vi "List Project Contents.vi"(11 "Selected Project":refnum<vi>) -> (3 "Selected Project Out":refnum<vi>)   [LabVIEW 2014]
doc: "<b>Controls:</b> \n<b>Inputs:</b>\n<b>Exit:</b>\n\n\n<b>Save Data to File:</b>\n\n\n<b>Selected Project:</b>\n\n\n<b>Tab Control:</b>\n\n\n<b>Re-Scan:</b>\n\n\n<b>Outputs:</b>\n<b>Project Name:</b>\n\n\n<b>Progress:</b>\n\n\n<b>Selected Project 2:</b>\n\n\n<b>Project Description:</b>"
uses:
  <userlib>/GA/VI Documentation Tool/TYPE_Version Status.ctl
  <vilib>/Utility/miscctls.llb/LVRowAndColumnTypeDef.ctl
  Type Defs/TYPE_Sorted Project Items.ctl
  Type Defs/TYPE_Project Summary.ctl
panel:
  out "Project Name":string caption="Project\nName"
  out "Project Description":string caption="Project\nDescription"
  in  "Tab Control":T1(tab)
  out "Summary":T2
  in  "Items List":i32[](listbox)
  out "Progress":i32(slide) caption="Sorting Project Items By Location" max=35
  in  "Re-Scan":bool
  in  "Save Data to File":bool
  in  "Exit":bool
  # "User.lib VIs Summary"
  # "Project VIs Summary"
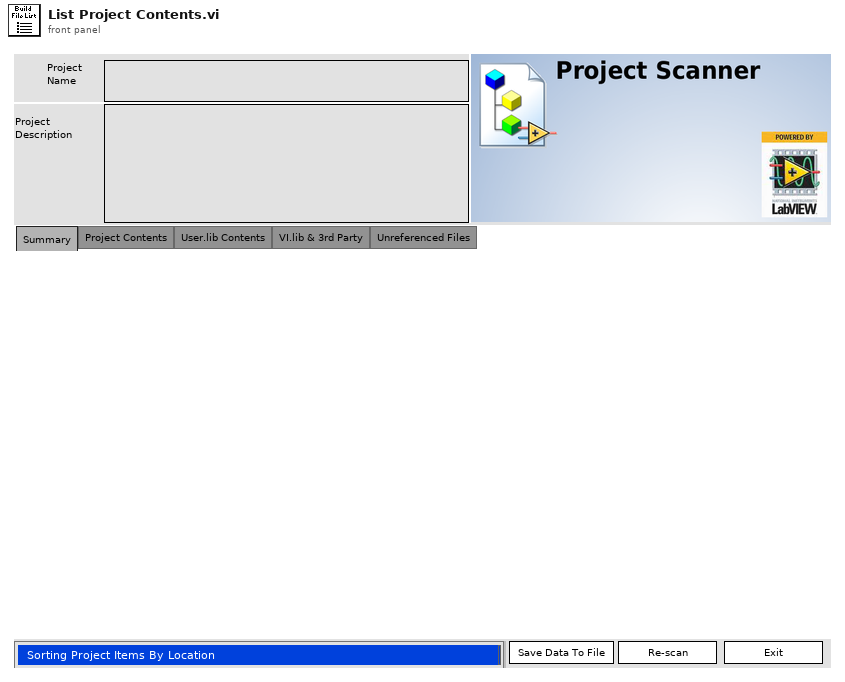
[diagram p1: front panel]
types:
  T1 = enum32{"Summary", "Project Contents", "User.lib Contents", "VI.lib & 3rd Party", "Unreferenced Files"}
  T2 = cluster{"Project Path":path, "Total VIs In Project":i32, "# of Unreviewed VIs":i32, "Date of Latest Reviewed VI":string, "# of VIs without Caller":i32, "#user.lib VIs":i32, "# of Unreviewed VIs (user.lib)":i32, "Review Date(user.lib)":string, "# withoutCaller(user.lib)":i32, "# of Modifed VIs":i32, "# of Modifed VIs (user.lib)":i32}
  T3 = enum32{"Invalid", "Standard", "Closed", "Hidden", "Minimized", "Maximized"}
  T4 = typedef "TYPE_Version Status.ctl" = enum16{"Development", "alpha", "beta", "Reviewed", "Bug", "Other"}
  T5 = typedef "LVRowAndColumnTypeDef.ctl" = cluster{"Row":i32, "Column":i32}
  T6 = enum32{"invalid app kind", "Development System", "Run Time System", "Student Edition", "Embedded LabVIEW", "Evaluation", "Custom"}
  T7 = typedef "TYPE_Sorted Project Items.ctl" = cluster{"VIs In Project":refnum<vi>[], "VIs In user.lib":refnum<vi>[], "VIs In vi.lib":refnum<vi>[]}
  T8 = typedef "TYPE_Project Summary.ctl" = cluster{"Project Name":string, "Project Path":path, "# VIs in Project":i32, "# VIs Unreviewed":i32, "Date of Last Review":timestamp, "# of VIs without Caller":i32, "Project Description":string, "# VIs Modified":i32}
  T9 = cluster{"Core":cluster{"Current VI Reference":refnum<vi>, "Close Panel on Exit?":bool}, "Selected Project":refnum<vi>, "Project Items":T7, "Project Summary":T8, "Project Member Data":string[][], "User.lib Member Data":string[][], "3rd Party Member Data":string[][], "Unref Files":path[]}
  T10 = typedef "TYPE_Description Cluster.ctl" = cluster{"VI Description":string, "VI Version":string, "Review Date":string, "Author":string, "Copyright":string, "Requirements Coverage":string}
  T11 = cluster{"Current VI Reference":refnum<vi>, "Close Panel on Exit?":bool}
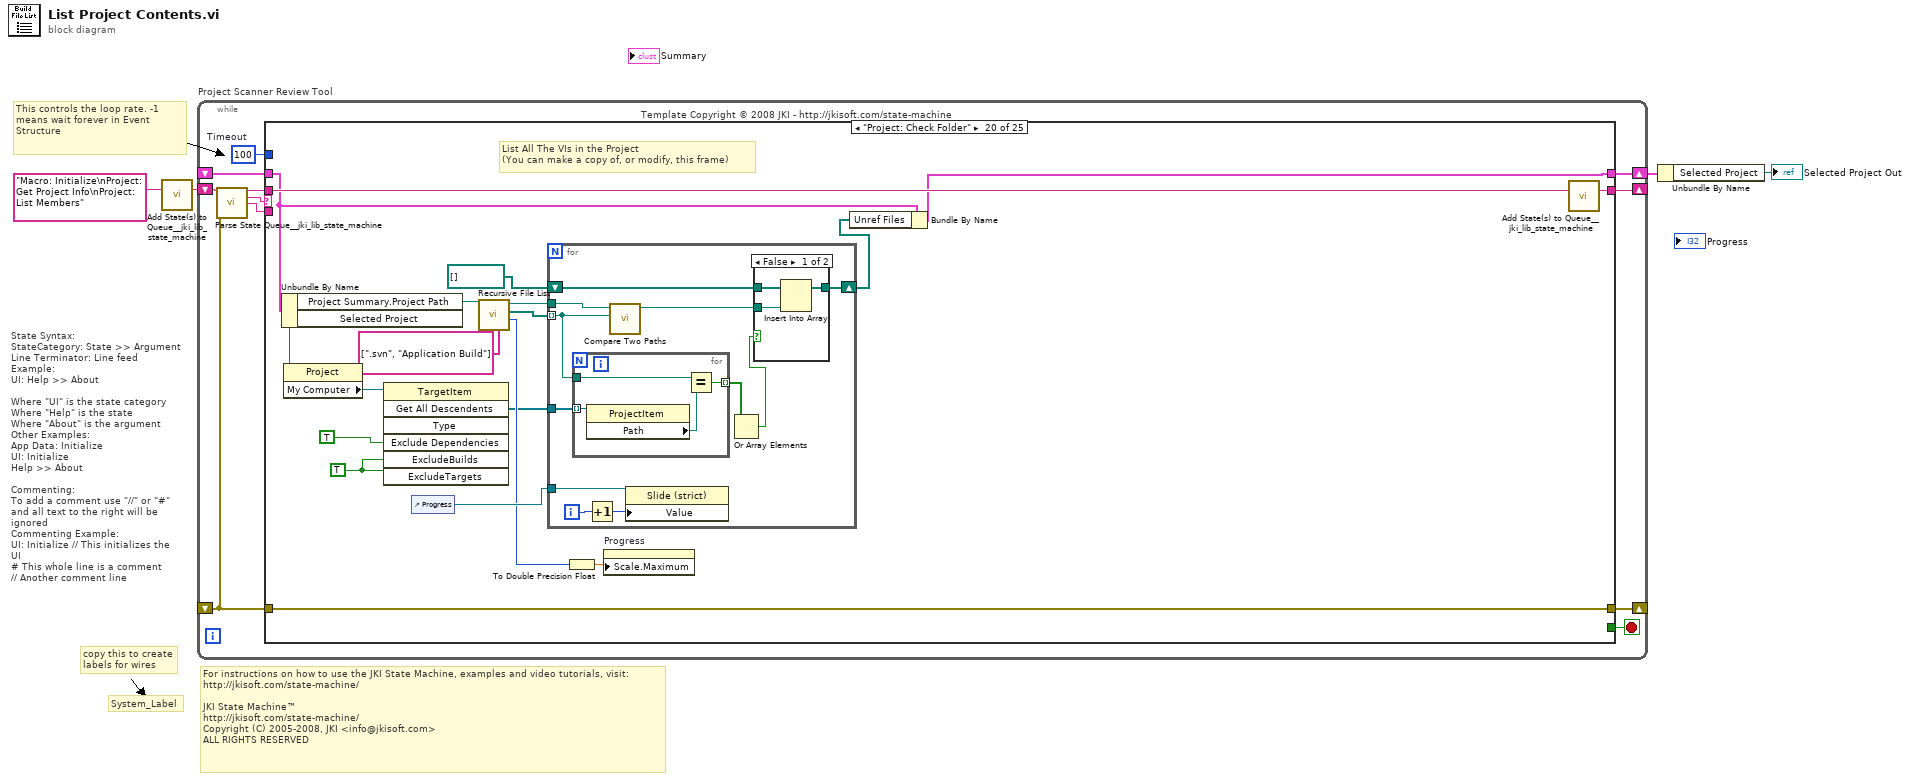
[diagram p0: block diagram]
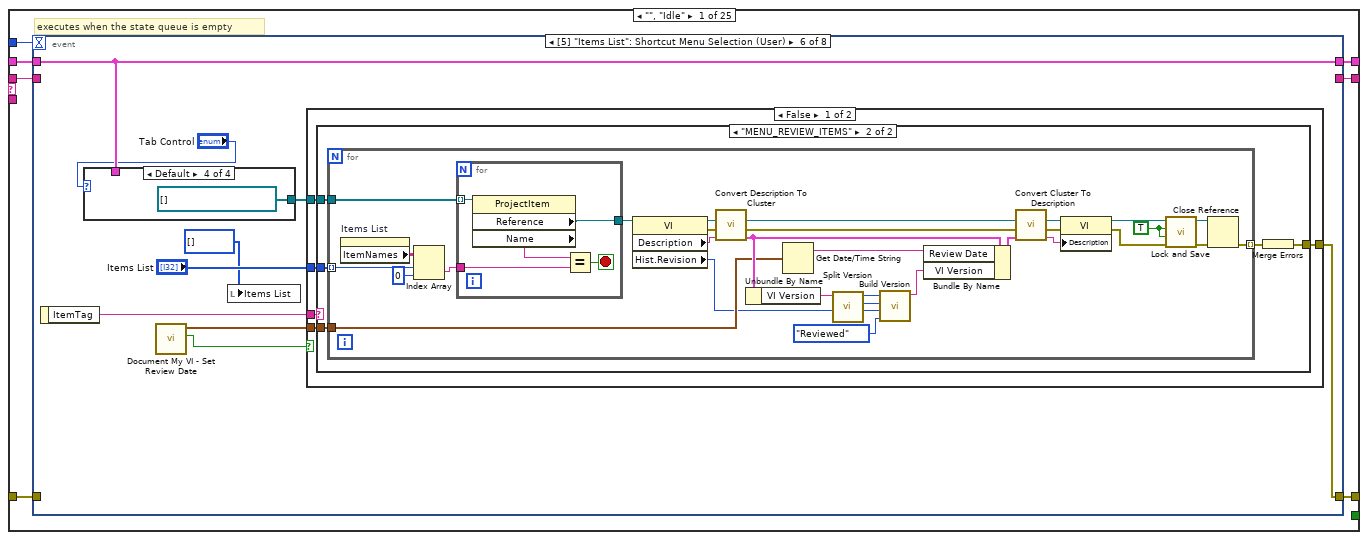
[diagram p2: hidden frame]
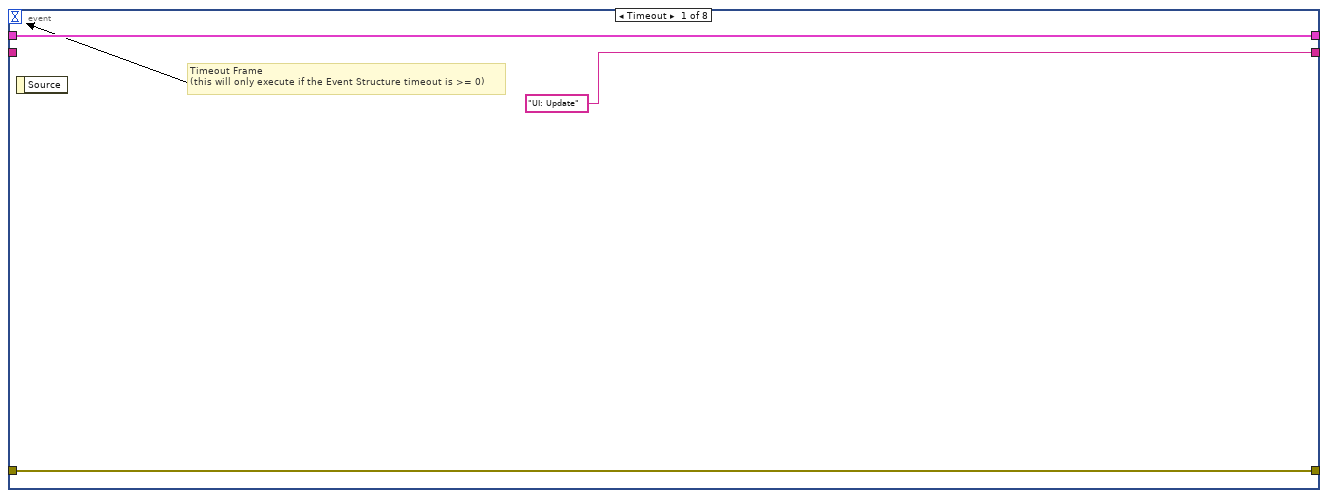
[diagram p3: hidden frame]
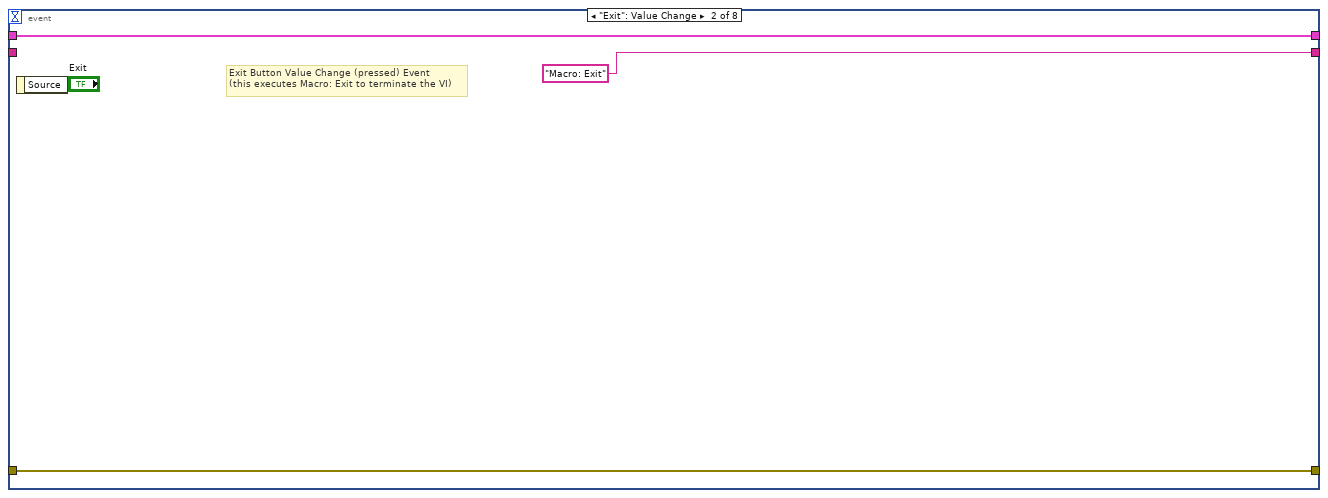
[diagram p4: hidden frame]
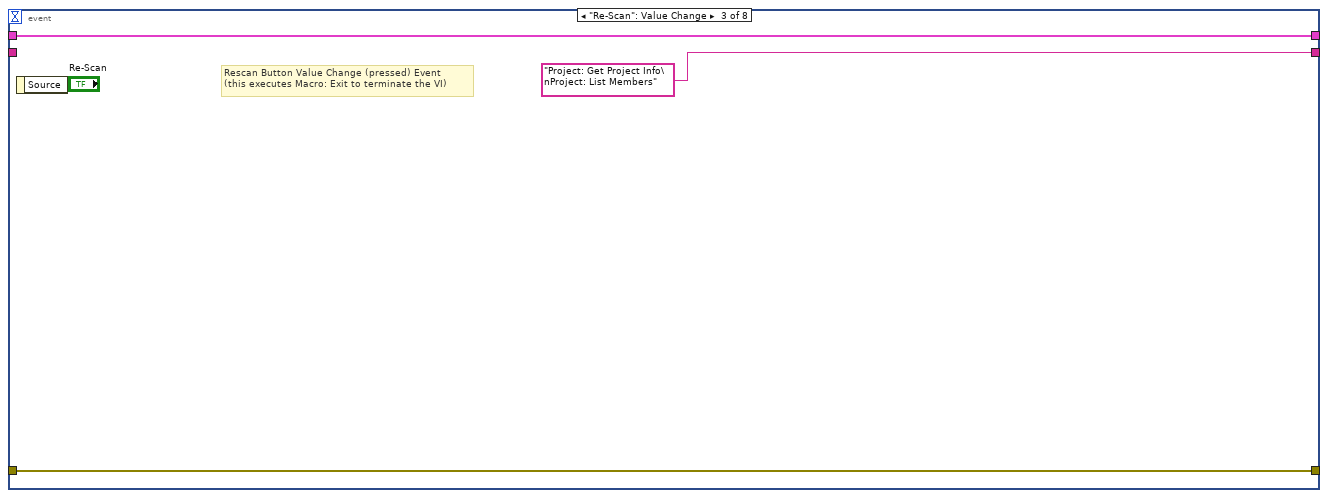
[diagram p5: hidden frame]
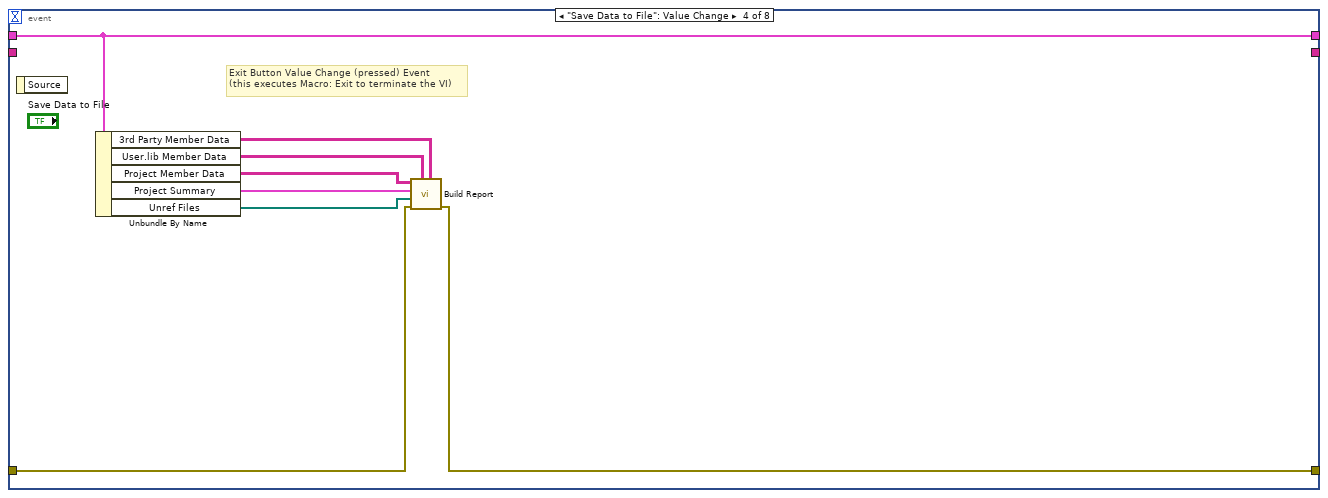
[diagram p6: hidden frame]
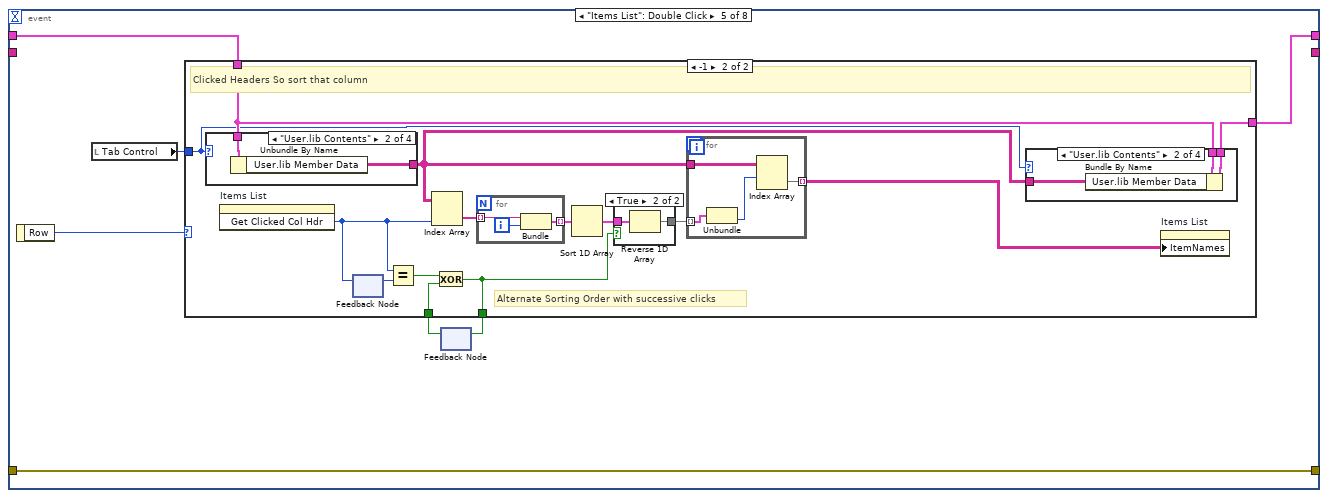
[diagram p7: hidden frame]
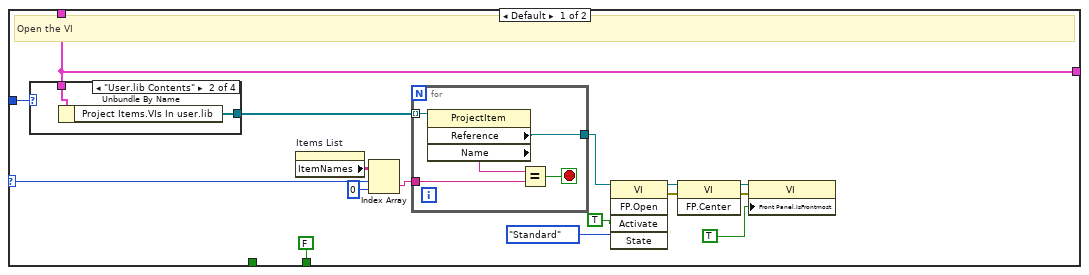
[diagram p8: hidden frame]
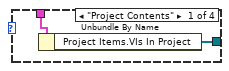
[diagram p9: hidden frame]
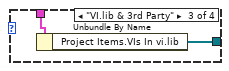
[diagram p10: hidden frame]
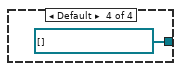
[diagram p11: hidden frame]
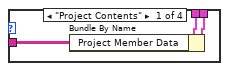
[diagram p13: hidden frame]
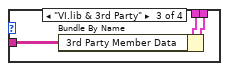
[diagram p14: hidden frame]
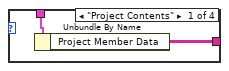
[diagram p16: hidden frame]
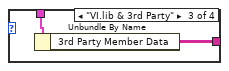
[diagram p17: hidden frame]
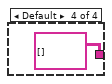
[diagram p18: hidden frame]
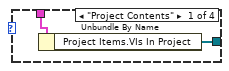
[diagram p19: hidden frame]
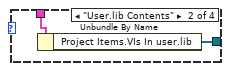
[diagram p20: hidden frame]
diagram:
  # "This controls the loop rate. -1 means wait forever in Event Structure"
  # "For instructions on how to use the JKI State Machine, examples and video tutorials, visit:\nhttp://jkisoft.com/state-machine/\n\nJKI State Machine™\nhttp://jkisoft.com/state-machine/\nCopyright (C) 2005-2008, JKI <info@jkisoft.com>\nALL RIGHTS RESERVED"
  # "State Syntax:\nStateCategory: State >> Argument\nLine Terminator: Line feed\nExample:\nUI: Help >> About\n\nWhere \"UI\" is the state category\nWhere \"Help\" is the state\nWhere \"About\" is the argument\nOther Examples:\nApp Data: Initialize\nUI: Initialize\nHelp >> About\n\nCommenting:\nTo add a comment use \"//\" or \"#\" and all text to the right will be ignored\nCommenting Example:\nUI: Initialize // This initializes the UI\n# This whole line is a comment\n// Another comment line"
  # "copy this to create labels for wires"
  # "System_Label"
  n1 = call <vilib>:"Add State(s) to Queue__jki_lib_state_machine.vi"("State(s) in (\"\")"="Macro: Initialize\nProject: Get Project Info\nProject: List Members") -> ("States Out"=w4:string)  [unwired: 14 in]
  n2 = while "Project Scanner Review Tool" {
    shift-right: [w8] -> w2
    shift-left: _ -> [w7]
    shift-right: [w11] -> _
    shift-left: _ -> [w5]
    shift-right: [w10] -> _
    shift-left: w4 -> [w12]
    stop <- w9 stop-if-true
    w6 = 100  # Timeout
    # "Template Copyright © 2008 JKI - http://jkisoft.com/state-machine"
    n3 = call <vilib>:"Parse State Queue__jki_lib_state_machine.vi"("State Queue"=w12, "Error In (no error)"=w5) -> ("Remaining States"=w14:string, "Current State"=w15:string, "Arguments"=w13:string)  [unwired: 11 in]
    n4 = case shown="\"Project: Check Folder\"" w15 {
      selector: w15 -> [_ _ w223 _ _ _ _ _ _ _ _ _ _ _ _ _ _ _ _ _ _ _ _ _ _]
      tunnel: w14 -> [w22 w222 w227 w239 w244 w256 w260 w272 w284 w288 w298 w303 w307 w313 w324 w357 w372 w376 w391 w421 w465 w486 w499 w514 w535]
      tunnel: w13 -> [_ _ _ _ _ _ _ _ _ _ _ _ _ w308 w318 _ _ _ _ _ _ _ _ _ _]
      tunnel: w7 -> [w20 w219 w225 w236 w242 w247 w257 w268 _ w285 w295 w300 w304 w311 w320 w355 w368 w373 w389 w405 w448 w479 w497 w512 w526]
      tunnel: [w19 w220 w229 errorcluster {"status"=FALSE, "code"=0, "source"=""} ("error out") w241 w253 w258 w262 w281 w286 w296 w301 w305 w309 w321 w352 w370 w374 w383 w417 w461 w480 w496 w508 w524] -> w11
      tunnel: w5 -> [w18 w220 w228 w235 w241 w253 w258 w266 w281 w286 w296 w301 w305 w310 w322 w353 w370 w374 w386 w417 w463 w480 w496 w509 w532]
      tunnel: [w21 w221 w226 w238 w243 w255 w259 w271 w283 w287 w297 w302 w306 w312 w323 w356 w371 w375 w390 w420 w464 w485 w498 w513 w534] -> w10
      tunnel: [_ _ _ _ TRUE _ _ _ _ _ _ _ _ _ _ _ _ _ _ _ _ _ _ _ _] -> w9
      tunnel: [w17 w219 w225 w236 w242 w254 w257 w268 w282 w285 w295 w300 w304 w311 w320 w355 w368 w373 w388 w404 w450 w478 w497 w511 w525] -> w8
      tunnel: w6 -> [w16 _ _ _ _ _ _ _ _ _ _ _ _ _ _ _ _ _ _ _ _ _ _ _ _]
      frame "", "Idle" {
        # "executes when the state queue is empty"
        n5 = event shown="[5] \"Items List\": Shortcut Menu Selection (User)" {
          selector: _ -> [_ _ _ _ _ _ _ _]
          dyn-events: _ -> [_ _ _ _ _ _ _ _]
          timeout: w16 -> [_ _ _ _ _ _ _ _]
          tunnel: w22 -> [_ _ _ _ _ _ _ _]
          tunnel: ["UI: Update" ("State(s) in Front (\"\")") "Macro: Exit" "Project: Get Project Info\nProject: List Members" _ _ _ _ "Macro: Exit"] -> w21
          tunnel: w20 -> [w24 w27 w30 w39 w43 w119 w176 w217]
          tunnel: [w25 w28 w31 w36 w46 w121 w175 w218] -> w19
          tunnel: w18 -> [w25 w28 w31 w37 w46 _ w175 w218]
          tunnel: [w24 w27 w30 w39 w42 w119 w176 w217] -> w17
          event Timeout {
            # "Timeout Frame\n(this will only execute if the Event Structure timeout is >= 0)"
            n6 = event-data() -> ()  [unwired: 1 in, 1 out]
          }
          event "Exit": Value Change {
            # "Exit Button Value Change (pressed) Event\n(this executes Macro: Exit to terminate the VI)"
            n7 = event-data() -> ()  [unwired: 1 in, 1 out]
          }
          event "Re-Scan": Value Change {
            # "Rescan Button Value Change (pressed) Event\n(this executes Macro: Exit to terminate the VI)"
            n8 = event-data() -> ()  [unwired: 1 in, 1 out]
          }
          event "Save Data to File": Value Change {
            # "Exit Button Value Change (pressed) Event\n(this executes Macro: Exit to terminate the VI)"
            n9 = event-data() -> ()  [unwired: 1 in, 1 out]
            n10 = Unbundle By Name(w39) -> ("3rd Party Member Data"=w33:string[][], "User.lib Member Data"=w34:string[][], "Project Member Data"=w35:string[][], "Project Summary"=w38:T8, "Unref Files"=w32:path[])
            n11 = call "Build Report.vi"("3rd Party Member Data"=w33, "User.lib Member Data"=w34, "error in (no error)"=w37, "Unreferenced Files"=w32, "Project Summary"=w38, "Project Member Data"=w35) -> ("error out"=w36:errorcluster)  [unwired: 5 in]
          }
          event "Items List": Double Click {
            n12 = event-data() -> ("Row"=w45:i32)  [unwired: 1 in]
            n13 = local read "Tab Control"() -> (w44:T1)
            n14 = feedback #1() -> (w40:bool)  [unwired: 1 in]
            n15 = case shown="-1" w45 {
              selector: w45 -> [w54 _]
              tunnel: w43 -> [w48 w88]
              tunnel: w44 -> [w49 w81]
              tunnel: [w48 w85] -> w42
              tunnel: [FALSE w75] -> w41
              tunnel: w40 -> [_ w77]
              frame Default {
                # "Open the VI"
                n16 = case shown="\"User.lib Contents\"" w49 {
                  tunnel: w48 -> [w64 w66 w68 _]
                  tunnel: [w63 w65 w67 refnum<vi>[] [] ("VIs In vi.lib")] -> w50
                  frame "Project Contents" {
                    n17 = Unbundle By Name(w64) -> ("Project Items.VIs In Project"=w63:refnum<vi>[])
                  }
                  frame "User.lib Contents" {
                    n18 = Unbundle By Name(w66) -> ("Project Items.VIs In user.lib"=w65:refnum<vi>[])
                  }
                  frame "VI.lib & 3rd Party" {
                    n19 = Unbundle By Name(w68) -> ("Project Items.VIs In vi.lib"=w67:refnum<vi>[])
                  }
                  frame Default {
                  }
                }
                n20 = property on="Items List" class="MCListbox (strict)"() -> ("ItemNames"=w55:string[][])  [unwired: 2 in, 2 out]
                n21 = Index Array(array=w55, index (row)=w54, index (col)=0 ("disabled index (col)")) -> (element=w51:string)
                n22 = for {
                  tunnel: [w74] -> w52
                  tunnel: w51 -> [w71]
                  tunnel: w50 -> [w73] mode=indexing
                  stop <- w70 stop-if-true
                  n23 = property class="ProjectItem"(reference=w73) -> ("Reference"=w74:refnum<vi>, "Name"=w72:string)  [unwired: 1 in, 2 out]
                  n24 = Equal?(x=w72, y=w71) -> (x = y?=w70:bool)
                }
                n25 = invoke class="VI" method="FP.Open"(reference=w52, "Activate"=TRUE ("Activate?"), "State"=T3."Standard") -> (reference out=w60:refnum<vi>, error out=w59:errorcluster)  [unwired: 2 in, 3 out]
                n26 = invoke class="VI" method="FP.Center"(reference=w60, error in=w59) -> (reference out=w58:refnum<vi>, error out=w57:errorcluster)  [unwired: 1 in, 1 out]
                n27 = property class="VI"(reference=w58, error in=w57, "Front Panel.IsFrontmost"=TRUE ("Front Panel Window:Is Frontmost")) -> ()  [unwired: 2 out]
              }
              frame -1 {
                # "Alternate Sorting Order with successive clicks"
                # "Clicked Headers So sort that column"
                n28 = case shown="\"User.lib Contents\"" w81 {
                  tunnel: w88 -> [w110 w112 w114 _]
                  tunnel: [w109 w111 w113 string[][] [] ("3rd Party Member Data")] -> w80
                  frame "Project Contents" {
                    n29 = Unbundle By Name(w110) -> ("Project Member Data"=w109:string[][])
                  }
                  frame "User.lib Contents" {
                    n30 = Unbundle By Name(w112) -> ("User.lib Member Data"=w111:string[][])
                  }
                  frame "VI.lib & 3rd Party" {
                    n31 = Unbundle By Name(w114) -> ("3rd Party Member Data"=w113:string[][])
                  }
                  frame Default {
                  }
                }
                n32 = invoke on="Items List" class="MCListbox (strict)" method="Get Clicked Col Hdr"() -> ("Get Clicked Column Header"=w83:i32)  [unwired: 3 in, 2 out]
                n33 = feedback-in #2(w83) -> ()
                n34 = feedback #2() -> (w84:i32)  [unwired: 1 in]
                n35 = Equal?(x=w83, y=w84) -> (x = y?=w76:bool)
                n36 = Index Array(array=w80, index (col)=w83) -> (element=w79:string[])  [unwired: 1 in]
                n37 = Exclusive Or(1:w77, 2:w76) -> (0:w75:bool)
                n38 = for {
                  tunnel: w79 -> [w90] mode=indexing
                  tunnel: [w89] -> w78 mode=indexing
                  i -> [w91]
                  n39 = Bundle(w90, w91) -> (w89:cluster{string, i32})  [unwired: 1 in]
                }
                n40 = Sort 1D Array(array=w78) -> (sorted array=w87:cluster{string, i32}[])
                n41 = case shown="True" w75 {
                  tunnel: w87 -> [w92 w94]
                  tunnel: [w92 w93] -> w82
                  frame False {
                  }
                  frame True {
                    n42 = Reverse 1D Array(array=w94) -> (reversed array=w93:cluster{string, i32}[])
                  }
                }
                n43 = for {
                  tunnel: w82 -> [w96] mode=indexing
                  tunnel: w80 -> [w98]
                  tunnel: [w97] -> w86 mode=indexing
                  n44 = Unbundle(w96) -> (w95:i32)  [unwired: 1 out]
                  n45 = Index Array(array=w98, index (row)=w95) -> (element=w97:string[])  [unwired: 1 in]
                }
                n46 = case shown="\"User.lib Contents\"" w81 {
                  tunnel: w88 -> [w101 w104 w107 w108]
                  tunnel: [w100 w103 w106 w108] -> w85
                  tunnel: w80 -> [w99 w102 w105 _]
                  frame "Project Contents" {
                    n47 = Bundle By Name(cluster=w101, "Project Member Data"=w99) -> (w100:T9)
                  }
                  frame "User.lib Contents" {
                    n48 = Bundle By Name(cluster=w104, "User.lib Member Data"=w102) -> (w103:T9)
                  }
                  frame "VI.lib & 3rd Party" {
                    n49 = Bundle By Name(cluster=w107, "3rd Party Member Data"=w105) -> (w106:T9)
                  }
                  frame Default {
                  }
                }
                n50 = property on="Items List" class="MCListbox (strict)"("ItemNames"=w86) -> ()  [unwired: 2 in, 2 out]
              }
            }
            n51 = feedback-in #1(w41) -> ()
          }
          event "Items List": Shortcut Menu Selection (User) {
            n52 = event-data() -> ("ItemTag"=w124:string)  [unwired: 1 in]
            n53 = case shown="Default" "Tab Control" {
              tunnel: w119 -> [w126 w128 w130 _]
              tunnel: [w125 w127 w129 refnum<vi>[] [] ("VIs In vi.lib")] -> w118
              frame "Project Contents" {
                n54 = Unbundle By Name(w126) -> ("Project Items.VIs In Project"=w125:refnum<vi>[])
              }
              frame "User.lib Contents" {
                n55 = Unbundle By Name(w128) -> ("Project Items.VIs In user.lib"=w127:refnum<vi>[])
              }
              frame "VI.lib & 3rd Party" {
                n56 = Unbundle By Name(w130) -> ("Project Items.VIs In vi.lib"=w129:refnum<vi>[])
              }
              frame Default {
              }
            }
            n57 = call <userlib>:"Document My VI - Set Review Date.vi"() -> ("Canceled"=w122:bool, "Date of Review out"=w123:timestamp)  [unwired: 9 in, 1 out]
            n58 = local write "Items List"(i32[] [] ("Items List")) -> ()
            n59 = case shown="False" w122 {
              tunnel: w124 -> [w136 _]
              tunnel: "Items List" -> [w135 _]
              tunnel: w123 -> [w134 _]
              tunnel: [w133 _] -> w121
              tunnel: w118 -> [w132 _]
              frame False {
                n60 = case shown="\"MENU_REVIEW_ITEMS\"" w136 {
                  tunnel: w135 -> [_ w141]
                  tunnel: w134 -> [_ w140]
                  tunnel: [_ w138] -> w133
                  tunnel: w132 -> [_ w137]
                  frame "False", Default {
                  }
                  frame "MENU_REVIEW_ITEMS" {
                    n61 = for {
                      tunnel: w141 -> [w166] mode=indexing
                      tunnel: w140 -> [w148]
                      tunnel: [w143] -> w139 mode=indexing
                      tunnel: w137 -> [w142]
                      w162 = TRUE ("Lock?")
                      n62 = property on="Items List" class="MCListbox (strict)"() -> ("ItemNames"=w169:string[][])  [unwired: 2 in, 2 out]
                      n63 = Index Array(array=w169, index (row)=w166, index (col)=0 ("disabled index (col)")) -> (element=w167:string)
                      n64 = for {
                        tunnel: [w174] -> w164
                        tunnel: w167 -> [w171]
                        tunnel: w142 -> [w173] mode=indexing
                        stop <- w170 stop-if-true
                        n65 = property class="ProjectItem"(reference=w173) -> ("Reference"=w174:refnum<vi>, "Name"=w172:string)  [unwired: 1 in, 2 out]
                        n66 = Equal?(x=w172, y=w171) -> (x = y?=w170:bool)
                      }
                      n67 = property class="VI"(reference=w164) -> (reference out=w149:refnum<vi>, error out=w165:errorcluster, "Description"=w163:string, "Hist.Revision"=w147:u32)  [unwired: 1 in]
                      n68 = call <userlib>:"Convert Description To Cluster.vi"("Description String (empty)"=w163, "error in (no error)"=w165) -> ("Description Cluster"=w150:T10, "error out"=w146:errorcluster)  [unwired: 8 in]
                      n69 = Unbundle By Name(w150) -> ("VI Version"=w156:string)
                      n70 = Get Date/Time String(seconds (now)=w148) -> (date string=w158:string)  [unwired: 2 in, 1 out]
                      n71 = call <userlib>:"Split Version.vi"("VI Version"=w156) -> ("Minor Version"=w155:u16, "Major Version"=w154:u16)  [unwired: 7 in, 2 out]
                      n72 = call <userlib>:"Build Version.vi"("Current Phase"=TYPE_Version_Status."Reviewed", "Revision"=w147, "Minor Revision"=w155, "Major Revision"=w154) -> ("VI Version"=w157:string)  [unwired: 7 in]
                      n73 = Bundle By Name(cluster=w150, "Review Date"=w158, "VI Version"=w157) -> (w153:T10)
                      n74 = call <userlib>:"Convert Cluster To Description.vi"("Description Cluster"=w153, "error in (no error)"=w146) -> ("Description String (empty)"=w152:string, "error out"=w151:errorcluster)  [unwired: 8 in]
                      n75 = property class="VI"(reference=w149, error in=w151, "Description"=w152) -> (reference out=w160:refnum<vi>, error out=w161:errorcluster)
                      n76 = call <userlib>:"Lock and Save.vi"("error in (no error)"=w161, "Revision Comments?"=w162, "Lock?"=w162, "VI Ref"=w160) -> ("error out"=w145:errorcluster, "VI Ref out"=w144:refnum<vi>)  [unwired: 6 in]
                      n77 = Close Reference(reference=w144, error in (no error)=w145) -> (error out=w143:errorcluster)
                    }
                    n78 = Merge Errors(w139) -> (w138:errorcluster)
                  }
                }
              }
              frame True {
              }
            }
          }
          event "Tab Control": Value Change {
            n79 = event-data() -> ("NewVal"=w177:T1)  [unwired: 1 in]
            n80 = case shown="\"Summary\"" w177 {
              selector: w177 -> [_ w184]
              tunnel: w176 -> [_ w183]
              frame "Summary" {
                n81 = property on="Summary" class="Clust (strict)"("Visible"=TRUE) -> ()  [unwired: 2 in, 2 out]
                n82 = property on="Items List" class="MCListbox (strict)"("Visible"=FALSE) -> ()  [unwired: 2 in, 2 out]
              }
              frame Default {
                n83 = property on="Summary" class="Clust (strict)"("Visible"=FALSE) -> ()  [unwired: 2 in, 2 out]
                n84 = case shown="\"Project Contents\"" w184 {
                  tunnel: w183 -> [w194 w198 w202 w209 _]
                  tunnel: [w193 w197 w201 w204 string[][] [] ("3rd Party Member Data")] -> w182
                  tunnel: [w192 w196 w200 w207 string[] [] ("Column Headers")] -> w181
                  tunnel: [u32[] [300, 125, 100, 75, 75, 300, 5000] u32[] [300, 125, 100, 75, 75, 300, 5000] u32[] [300, 3000] u32[] [5000] u32[] [5000]] -> w180
                  frame "Project Contents" {
                    w192 = string[] ["VI Name", "VI Version", "Review Date", "Review?", "# of Callers", "Relative Path", "Actions/Comments/Questions"]  # Column Headers
                    n85 = Unbundle By Name(w194) -> ("Project Member Data"=w193:string[][])
                  }
                  frame "User.lib Contents" {
                    w196 = string[] ["VI Name", "VI Version", "Review Date", "Review?", "# of Callers", "Relative Path", "Actions/Comments/Questions"]  # Column Headers
                    n86 = Unbundle By Name(w198) -> ("User.lib Member Data"=w197:string[][])
                  }
                  frame "VI.lib & 3rd Party" {
                    w200 = string[] ["VI Name", "VI File Path"]  # Column Headers
                    n87 = Unbundle By Name(w202) -> ("3rd Party Member Data"=w201:string[][])
                  }
                  frame "Unreferenced Files" {
                    w207 = string[] ["VI Name"]  # Column Headers
                    n88 = Unbundle By Name(w209) -> ("Unref Files"=w208:path[])
                    n89 = for {
                      tunnel: w208 -> [w211] mode=indexing
                      tunnel: [w210] -> w206 mode=indexing
                      n90 = Strip Path(path=w211) -> (name=w210:string)  [unwired: 1 out]
                    }
                    n91 = Build Array(w206) -> (w205:string[][])
                    n92 = Transpose 2D Array(2D array=w205) -> (transposed array=w204:string[][])
                  }
                  frame "Summary" {
                  }
                }
                n93 = property on="Items List" class="MCListbox (strict)"("Visible"=TRUE, "ItemNames"=w182, "ColHdrString"=w181) -> ()  [unwired: 2 in, 2 out]
                n94 = for {
                  tunnel: w180 -> [w187] mode=indexing
                  i -> [w188]
                  n95 = Bundle(cluster=T5 {"Row"=0, "Column"=0} ("Active Cell:Active Cell"), "Column"=w188) -> (w189:T5)  [unwired: 1 in]
                  n96 = property on="Items List" class="MCListbox (strict)"("ActiveCell"=w189, "Width"=w187) -> ()  [unwired: 2 in, 2 out]
                }
              }
            }
          }
          event Panel Close? {
            # "Discard the event because we'll close the front panel ourselves in Macro: Exit"
            # "Close Panel button (pressed) Event\n(this executes Macro: Exit to terminate the VI)"
            n97 = event-data() -> ()  [unwired: 1 in, 1 out]
            n98 = event-data("Discard?"=TRUE) -> ()  [unwired: 1 in, 1 out]
          }
        }
      }
      frame "---------- Core ----------" {
        # "Do not put any code in this frame.\n(it is a separator no-op)"
        n99 = call <vilib>:"Add State(s) to Queue__jki_lib_state_machine.vi"("State(s) in (\"\")"=w222) -> ("States Out"=w221:string)  [unwired: 14 in]
      }
      frame Default {
        w232 = 42 items=["No error", "Argument error", "Memory is full", "Out of zone", "End of file", "File already open", "Generic file I/O error", "File not found", "File permission error", "Disk is full", "Duplicate path", "Too many files open", "System feature not enabled", "Resource file not found", "Cannot add resource", "Resource not found", "Image not found", "Image memory error", "Pen does not exist", "Config type invalid", "Config token not found", "Config parse error", "Config memory error", "Bad external code format", "Bad external code offset", "External code not present", "Null window", "Destroy window error", "Null menu", "Print aborted", "Bad print record", "Print driver error", "Windows error during printing", "Memory error during printing", "Print dialog error", "Generic print error", "Invalid device refnum", "Device not found", "Device parameter error", "Device unit error", "Cannot open device", "Device call aborted", "Generic error", "Cancelled by user", "Object ID too low", "Object ID too high", "Object not in heap", "Unknown heap", "Unknown object (invalid DefProc)", "Unknown object (DefProc not in table)", "Message out of range", "Invalid (null) method", "Unknown message", "Manager call not supported", "Bad address", "Network operation in progress", "Network operation timed out", "Connection is busy", "Network attribute not supported", "Network error", "Address in use", "System out of memory", "Connection aborted", "Connection refused", "Not connected", "Already connected", "Connection closed", "Initialization error (interapplication manager)", "Bad occurrence", "Wait on unbound occurrence handler", "Occurrence queue overflow", "Datalog type conflict", "Unused", "Unrecognized type (interapplication manager)", "Memory corrupt", "Failed to make temporary DLL", "Old CIN version", "Drag socket not found", "Failed to load drop-object", "Failed to register OLE object", "Failed to release OLE object", "Format specifier type mismatch", "Unknown format specifier", "Too few format specifiers", "Too many format specifiers", "Scan failed", "Newer CIN version", "Error converting to variant", "Runtime menu error", "Password tampered", "Variant attribute not found", "Incompatible variant data type", "Event data is not available", "Event Store is not present", "Occurrence is not found", "Event Queue is not created", "Event info is not available", "Refnum passed is NULL", "Error retrieving Class GUID", "Error retrieving CoClass GUID", "Error retrieving TypeLib GUID.", "Bad built application magic bytes.", "Specific driver is different from the specific driver associated with the Logical Name.", "There is no session opened to the class driver.", "Max Error", "MAX - Error with config objects", "MAX - Error loading configuration", "MAX - Group not supported"]
        # "Current State"
        # "Do not delete, rename, or modify this frame.\n(this is used to capture unhandled states and typos)"
        # "Handle mistyped state name (developer tool)"
        n100 = Format Into String(format string="Software Exception: Unhandled State \"%s\"." ("message"), error in=w228, w223) -> (resulting string=w231:string, error out=w230:errorcluster)  [unwired: 1 in]
        n101 = call <vilib>:"Error Cluster From Error Code.vi"("show call chain? (False)"=TRUE, "error in (no error)"=w230, "error message (\"\")"=w231, "error code (0)"=w232) -> ("error out"=w229:errorcluster)  [unwired: 5 in]
        n102 = call <vilib>:"Add State(s) to Queue__jki_lib_state_machine.vi"("State(s) in (\"\")"=w227) -> ("States Out"=w226:string)  [unwired: 14 in]
      }
      frame "Error Handler" {
        # "Unhandled Error -- Display it"
        # "Handle any errors here.\nYou can also output any states to clean-up after errors occur"
        # "Clear error"
        n103 = call <vilib>:"General Error Handler.vi"("error in (no error)"=w235) -> ()  [unwired: 10 in, 5 out]
        n104 = call <vilib>:"Add State(s) to Queue__jki_lib_state_machine.vi"("State(s) in Front (\"\")"="/* Post Error States", "State(s) in (\"\")"=w239) -> ("States Out"=w238:string)  [unwired: 13 in]
      }
      frame "Exit" {
        # "Do not put any code in this frame.\n(No errors that occur here will be handled.)"
        n105 = call <vilib>:"Add State(s) to Queue__jki_lib_state_machine.vi"("State(s) in (\"\")"=w244) -> ("States Out"=w243:string)  [unwired: 14 in]
      }
      frame "Initialize Core Data" {
        # "Do not delete, rename, or modify this frame.\n(this is used to determine panel behavior on exit)"
        # "originally closed?"
        # "exe?"
        # "If panel starts closed or is an EXE, then close it when we exit"
        n106 = property class="VI"() -> ("Front Panel.Open"=w252:bool)  [unwired: 2 in, 2 out]
        n107 = property class="App"() -> ("App.Kind"=w251:T6)  [unwired: 2 in, 2 out]
        n108 = control-ref of="Current VI Reference"() -> (w245:refnum<vi>)
        n109 = Not(x=w252) -> (.not. x?=w249:bool)
        n110 = Equal?(x=w251, y=T6."Run Time System" ("Application:Kind")) -> (x = y?=w248:bool)
        n111 = Or(x=w249, y=w248) -> (x .or. y?=w246:bool)
        n112 = Bundle By Name(cluster=w247, "Core.Current VI Reference"=w245, "Core.Close Panel on Exit?"=w246) -> (w254:T9)
        n113 = call <vilib>:"Add State(s) to Queue__jki_lib_state_machine.vi"("State(s) in (\"\")"=w256) -> ("States Out"=w255:string)  [unwired: 14 in]
      }
      frame "---------- Data ----------" {
        # "Do not put any code in this frame.\n(It is a separator no-op. You can make a copy of this frame to create a new Data frame)"
        n114 = call <vilib>:"Add State(s) to Queue__jki_lib_state_machine.vi"("State(s) in (\"\")"=w260) -> ("States Out"=w259:string)  [unwired: 14 in]
      }
      frame "Data: Cleanup" {
        w261 = 1055  # Code to Clear (0)
        # "Cleanup any data and references, here.\n(this is called automatically, by the Macro: Exit)"
        n115 = Unbundle By Name(w268) -> ("Core.Current VI Reference"=w270:refnum<vi>, "Selected Project"=w263:refnum<vi>, "Selected Project"=w264:refnum<vi>)
        n116 = Close Reference(reference=w264, error in (no error)=w266) -> (error out=w267:errorcluster)
        n117 = Close Reference(reference=w263, error in (no error)=w267) -> (error out=w265:errorcluster)
        n118 = Close Reference(reference=w270, error in (no error)=w265) -> (error out=w269:errorcluster)
        n119 = call <vilib>:"Clear Errors.vi"("error in (no error)"=w269, "specific error code to clear (0: all)"=w261) -> ("error out"=w262:errorcluster)  [unwired: 4 in, 1 out]
        n120 = call <vilib>:"Add State(s) to Queue__jki_lib_state_machine.vi"("State(s) in (\"\")"=w272) -> ("States Out"=w271:string)  [unwired: 14 in]
      }
      frame "Data: Initialize" {
        w273 = path[] []  # Unref Files
        w274 = string[][] []  # 3rd Party Member Data
        w275 = string[][] []  # User.lib Member Data
        w277 = T8 {"Project Name"="", "Project Path"=path "", "# VIs in Project"=0, "# VIs Unreviewed"=0, "Date of Last Review"=timestamp(0 s since 1904-01-01), "# of VIs without Caller"=0, "Project Description"="", "# VIs Modified"=0}  # Project Summary
        w276 = T7 {"VIs In Project"=[], "VIs In user.lib"=[], "VIs In vi.lib"=[]}  # Project Items
        w278 = string[][] []  # Project Member Data
        w280 = T11 {"Current VI Reference"=refnum, "Close Panel on Exit?"=FALSE}  # Core
        # "do not delete - used by framework"
        # "Data names and types of shift register data are defined by this bundle."
        # "Initialize the shift-register data, here.\n(data names are defined by what you wire into the bundle function)"
        n121 = Bundle("Core"=w280, "Selected Project"="Selected Project", "Project Items"=w276, "Project Summary"=w277, "Project Member Data"=w278, "User.lib Member Data"=w275, "3rd Party Member Data"=w274, "Unref Files"=w273) -> (w282:T9)  [unwired: 1 in]
        n122 = call <vilib>:"Add State(s) to Queue__jki_lib_state_machine.vi"("State(s) in (\"\")"=w284) -> ("States Out"=w283:string)  [unwired: 14 in]
      }
      frame "---------- Macro ----------" {
        # "Do not put any code in this frame.\n(It is a separator no-op. You can make a copy of this frame to create a new Macro frame)"
        n123 = call <vilib>:"Add State(s) to Queue__jki_lib_state_machine.vi"("State(s) in (\"\")"=w288) -> ("States Out"=w287:string)  [unwired: 14 in]
      }
      frame "Macro: Exit" {
        # "Exit Macro\n(This is called once, when the VI exits)"
        n124 = Unbundle By Name(w295) -> ("Core.Close Panel on Exit?"=w294:bool)
        n125 = Select(t="UI: Front Panel State >> Close", s=w294, f="") -> (s? t:f=w291:string)
        n126 = call <vilib>:"Add State(s) to Queue__jki_lib_state_machine.vi"("State(s) in (\"\")"=w291, "State(s) at Back (\"\")"="Data: Cleanup\nExit") -> ("States Out"=w289:string)  [unwired: 13 in]
        n127 = call <vilib>:"Add State(s) to Queue__jki_lib_state_machine.vi"("State(s) in Front (\"\")"=w289, "State(s) in (\"\")"=w298) -> ("States Out"=w297:string)  [unwired: 13 in]
      }
      frame "Macro: Initialize" {
        w299 = "Data: Initialize\nInitialize Core Data\nUI: Initialize\nUI: Front Panel State >> Open"  # Data: Initialize Initialize Core Data UI: Initialize UI: Front Panel State >> Open
        # "Initialization Macro\n(This is called once, when the VI starts)"
        n128 = call <vilib>:"Add State(s) to Queue__jki_lib_state_machine.vi"("State(s) in Front (\"\")"=w299, "State(s) in (\"\")"=w303) -> ("States Out"=w302:string)  [unwired: 13 in]
      }
      frame "---------- UI ----------" {
        # "Do not put any code in this frame.\n(It is a separator no-op. You can make a copy of this frame to create a new UI frame)"
        n129 = call <vilib>:"Add State(s) to Queue__jki_lib_state_machine.vi"("State(s) in (\"\")"=w307) -> ("States Out"=w306:string)  [unwired: 14 in]
      }
      frame "UI: Cursor Set" {
        # "Argument"
        # "Set and Unset Cursor Busy.\n(Usage: \"UI: Cursor Set >> Busy|Idle\")"
        n130 = case shown="\"Idle\", Default" w308 {
          tunnel: w310 -> [w315 w317]
          tunnel: [w314 w316] -> w309
          frame "Idle", Default {
            n131 = call <vilib>:"Unset Busy.vi"("error in (no error)"=w315) -> ("error out"=w314:errorcluster)  [unwired: 10 in]
          }
          frame "Busy" {
            n132 = call <vilib>:"Set Busy.vi"("error in (no error)"=w317) -> ("error out"=w316:errorcluster)  [unwired: 9 in, 1 out]
          }
        }
        n133 = call <vilib>:"Add State(s) to Queue__jki_lib_state_machine.vi"("State(s) in (\"\")"=w313) -> ("States Out"=w312:string)  [unwired: 14 in]
      }
      frame "UI: Front Panel State" {
        # "Argument"
        # "Set Front Panel Open or Closed\n(Usage: \"UI: Front Panel State >> Open|Close\")"
        n134 = Unbundle By Name(w320) -> ("Core.Current VI Reference"=w319:refnum<vi>)
        n135 = case shown="\"Open\", Default" w318 {
          tunnel: w322 -> [w328 w341]
          tunnel: [w330 w342] -> w321
          tunnel: w319 -> [w329 w339]
          frame "Open", Default {
            n136 = property class="VI"(reference=w329, error in=w328) -> (reference out=w326:refnum<vi>, error out=w327:errorcluster, "Front Panel.Open"=w325:bool)
            n137 = case shown="True" w325 {
              tunnel: [w333 w336] -> w330
              tunnel: w327 -> [w332 w336]
              tunnel: w326 -> [w331 _]
              frame False {
                n138 = invoke class="VI" method="FP.Open"(reference=w331, error in=w332, "Activate"=TRUE, "State"=T3."Standard") -> (error out=w333:errorcluster)  [unwired: 1 in, 4 out]
              }
              frame True {
              }
            }
          }
          frame "Close" {
            n139 = property class="VI"(reference=w339, error in=w341) -> (reference out=w338:refnum<vi>, error out=w340:errorcluster, "Front Panel.Open"=w337:bool)
            n140 = case shown="True" w337 {
              tunnel: [w343 w346] -> w342
              tunnel: w340 -> [w343 w345]
              tunnel: w338 -> [_ w344]
              frame False {
              }
              frame True {
                n141 = invoke class="VI" method="FP.Close"(reference=w344, error in=w345) -> (error out=w346:errorcluster)  [unwired: 1 in, 2 out]
              }
            }
          }
        }
        n142 = call <vilib>:"Add State(s) to Queue__jki_lib_state_machine.vi"("State(s) in (\"\")"=w324) -> ("States Out"=w323:string)  [unwired: 14 in]
      }
      frame "UI: Initialize" {
        # "Initialize the User Interface, here.\n(this is called automatically, by the Macro: Init)"
        n143 = Unbundle By Name(w355) -> ("Core.Current VI Reference"=w354:refnum<vi>)
        n144 = property on="Summary" class="Clust (strict)"("Visible"=FALSE) -> ()  [unwired: 2 in, 2 out]
        n145 = invoke class="VI" method="Default Vals.Reinit All"(reference=w354, error in=w353) -> (error out=w352:errorcluster)  [unwired: 1 in, 2 out]
        n146 = property on="Items List" class="MCListbox (strict)"("Visible"=FALSE, "ItemNames"=string[][] [] ("Item Names"), "ActiveCell"=T5 {"Row"=0, "Column"=0} ("Active Cell:Active Cell"), "Width"=u32 5000 ("Active Cell:Cell Size:Width")) -> ()  [unwired: 2 in, 2 out]
        n147 = call <vilib>:"Add State(s) to Queue__jki_lib_state_machine.vi"("State(s) in (\"\")"=w357) -> ("States Out"=w356:string)  [unwired: 14 in]
      }
      frame "UI: Update" {
        # "Update the User Interface, here.\n(this is called automatically, by the Timeout event)"
        n148 = Unbundle By Name(w368) -> ("Project Summary.Project Name"=→"Project Name":string, "Project Summary.Project Path"=w363:path, "Project Summary.# VIs in Project"=w362:i32, "Project Summary.# VIs Unreviewed"=w361:i32, "Project Summary.Date of Last Review"=w366:timestamp, "Project Summary.# of VIs without Caller"=w359:i32, "Project Summary.Project Description"=→"Project Description":string, "Project Summary.# VIs Modified"=w358:i32)
        n149 = Get Date/Time String(seconds (now)=w366) -> (date string=w360:string)  [unwired: 2 in, 1 out]
        n150 = local read "Summary"() -> (w364:T2)
        n151 = Bundle By Name(cluster=w364, "Project Path"=w363, "Total VIs In Project"=w362, "# of Unreviewed VIs"=w361, "Date of Latest Reviewed VI"=w360, "# of VIs without Caller"=w359, "# of Modifed VIs"=w358) -> (w365:T2)
        n152 = local write "Summary"(w365) -> ()
        n153 = call <vilib>:"Add State(s) to Queue__jki_lib_state_machine.vi"("State(s) in (\"\")"=w372) -> ("States Out"=w371:string)  [unwired: 14 in]
      }
      frame "---------- Projects ----------" {
        # "Template Separator\n(You can make a copy of, or modify, this frame)"
        n154 = call <vilib>:"Add State(s) to Queue__jki_lib_state_machine.vi"("State(s) in (\"\")"=w376) -> ("States Out"=w375:string)  [unwired: 14 in]
      }
      frame "Project: Get Member Info" {
        # "List All The VIs in the Project\n(You can make a copy of, or modify, this frame)"
        n155 = Unbundle By Name(w389) -> ("Project Summary"=w381:T8, "Project Summary.Project Path"=w387:path, "Project Member Data"=w385:string[][], "Project Items.VIs In Project"=w377:refnum<vi>[])
        n156 = control-ref of="Progress"() -> (w384:refnum<vi>)
        n157 = for {
          tunnel: w387 -> [w402]
          tunnel: w377 -> [w397] mode=indexing
          shift-right: [w399] -> w383
          shift-left: w386 -> [w400]
          shift-right: [w401] -> w382
          shift-left: w385 -> [w398]
          tunnel: w384 -> [w395]
          i -> [w394]
          n158 = property class="ProjectItem"(reference=w397) -> ("Reference"=w396:refnum<vi>)  [unwired: 1 in, 2 out]
          n159 = Increment(x=w394) -> (x+1=w393:i32)
          n160 = property on="Property Node" class="Slide (strict)"(reference=w395, "Value"=w393) -> (reference out=w392:refnum<vi>)  [unwired: 1 in, 1 out]
          n161 = call "Scan Project Items.vi"("Slide in"=w392, "Project Path"=w402, "error in (no error)"=w400, "VI Refnum"=w396, "Member Data in"=w398) -> ("error out"=w399:errorcluster, "Member Data out"=w401:string[][])  [unwired: 5 in]
        }
        n162 = Array Size(array=w377) -> (size(s)=w378:i32)
        n163 = To Double Precision Float(number=w378) -> (double precision float=w379:dbl)
        n164 = property on="Progress" class="Slide (strict)"("Scale.Maximum"=w379) -> ()  [unwired: 2 in, 2 out]
        n165 = call "Summarize Project Items.vi"("Member Data"=w382, "Project Summary"=w381) -> ("Project Summary Out"=w380:T8)  [unwired: 9 in]
        n166 = Bundle By Name(cluster=w389, "Project Summary"=w380, "Project Member Data"=w382) -> (w388:T9)
        n167 = call <vilib>:"Add State(s) to Queue__jki_lib_state_machine.vi"("State(s) in (\"\")"=w391) -> ("States Out"=w390:string)  [unwired: 14 in]
      }
      frame "Project: Check Folder" {
        w411 = TRUE ("ExcludeDependencies")
        # "List All The VIs in the Project\n(You can make a copy of, or modify, this frame)"
        n168 = Unbundle By Name(w405) -> ("Project Summary.Project Path"=w416:path, "Selected Project"=w409:refnum<vi>)
        n169 = property class="Project"(reference=w409) -> ("My Computer"=w412:refnum<vi>)  [unwired: 1 in, 2 out]
        n170 = invoke class="TargetItem" method="Get All Descendents"(reference=w412, "Exclude Dependencies"=TRUE ("ExcludeDependencies"), "ExcludeBuilds"=w411, "ExcludeTargets"=w411) -> ("All Descendents"=w408:refnum<vi>[])  [unwired: 3 in, 6 out]
        n171 = control-ref of="Progress"() -> (w419:refnum<vi>)
        n172 = call <vilib>:"Recursive File List.vi"("Folders to Exclude"=string[] [".svn", "Application Build"], "Folder Path"=w416) -> ("Number of Files"=w415:i32, "All Files in Dir"=w414:path[], "dup Folder Path"=w406:path)  [unwired: 5 in, 2 out]
        n173 = for {
          tunnel: w408 -> [w432]
          tunnel: w419 -> [w431]
          tunnel: w414 -> [w423] mode=indexing
          shift-right: [w428] -> w403
          shift-left: path[] [] ("All Files in Dir") -> [w427]
          tunnel: w406 -> [w424]
          i -> [w430]
          n174 = for {
            tunnel: w432 -> [w440] mode=indexing
            tunnel: w423 -> [w438]
            tunnel: [w437] -> w426 mode=indexing
            n175 = property class="ProjectItem"(reference=w440) -> ("Path"=w439:path)  [unwired: 1 in, 2 out]
            n176 = Equal?(x=w438, y=w439) -> (x = y?=w437:bool)
          }
          n177 = Increment(x=w430) -> (x+1=w429:i32)
          n178 = call <vilib>:"Compare Two Paths.vi"("Path 2"=w423, "Path 1"=w424) -> ("Relative Path from 1 to 2"=w422:path)  [unwired: 6 in, 3 out]
          n179 = property on="Property Node" class="Slide (strict)"(reference=w431, "Value"=w429) -> ()  [unwired: 1 in, 2 out]
          n180 = Or Array Elements(Boolean array=w426) -> (logical OR=w425:bool)
          n181 = case shown="False" w425 {
            tunnel: [w435 w436] -> w428
            tunnel: w427 -> [w434 w436]
            tunnel: w422 -> [w433 _]
            frame False {
              n182 = Insert Into Array(array=w434, new element=w433) -> (w435:path[])  [unwired: 1 in]
            }
            frame True {
            }
          }
        }
        n183 = To Double Precision Float(number=w415) -> (double precision float=w418:dbl)
        n184 = property on="Progress" class="Slide (strict)"("Scale.Maximum"=w418) -> ()  [unwired: 2 in, 2 out]
        n185 = Bundle By Name(cluster=w405, "Unref Files"=w403) -> (w404:T9)
        n186 = call <vilib>:"Add State(s) to Queue__jki_lib_state_machine.vi"("State(s) in (\"\")"=w421) -> ("States Out"=w420:string)  [unwired: 14 in]
      }
      frame "User.lib:  Get Info" {
        # "List All The VIs in the Project\n(You can make a copy of, or modify, this frame)"
        n187 = Unbundle By Name(w448) -> ("Project Items.VIs In user.lib"=w452:refnum<vi>[])
        n188 = VI Library() -> (path=w455:path)
        n189 = control-ref of="Progress"() -> (w462:refnum<vi>)
        n190 = Array Size(array=w452) -> (size(s)=w453:i32)
        n191 = Strip Path(path=w455) -> (stripped path=w457:path)  [unwired: 1 out]
        n192 = To Double Precision Float(number=w453) -> (double precision float=w454:dbl)
        n193 = Build Path(base path=w457, name or relative path="user.lib") -> (appended path=w451:path)
        n194 = for {
          tunnel: w451 -> [w476]
          tunnel: w452 -> [w471] mode=indexing
          shift-right: [w473] -> w461
          shift-left: w463 -> [w474]
          shift-right: [w475] -> w449
          shift-left: string[][] [] ("Member Data out") -> [w472]
          tunnel: w462 -> [w468]
          i -> [w466]
          n195 = property class="ProjectItem"(reference=w471) -> ("Reference"=w470:refnum<vi>)  [unwired: 1 in, 2 out]
          n196 = Increment(x=w466) -> (x+1=w469:i32)
          n197 = property on="Property Node" class="Slide (strict)"(reference=w468, "Value"=w469) -> (reference out=w467:refnum<vi>)  [unwired: 1 in, 1 out]
          n198 = call "Scan Project Items.vi"("Slide in"=w467, "Project Path"=w476, "error in (no error)"=w474, "VI Refnum"=w470, "Member Data in"=w472) -> ("error out"=w473:errorcluster, "Member Data out"=w475:string[][])  [unwired: 5 in]
        }
        n199 = property on="Progress" class="Slide (strict)"("Scale.Maximum"=w454) -> ()  [unwired: 2 in, 2 out]
        n200 = call "Summarize Project Items.vi"("Member Data"=w449) -> ("Project Summary Out"=w460:T8)  [unwired: 10 in]
        n201 = Unbundle By Name(w460) -> ("# VIs in Project"=w445:i32, "# VIs Unreviewed"=w444:i32, "Date of Last Review"=w459:timestamp, "# of VIs without Caller"=w442:i32, "# VIs Modified"=w441:i32)
        n202 = Bundle By Name(cluster=w448, "User.lib Member Data"=w449) -> (w450:T9)
        n203 = Get Date/Time String(seconds (now)=w459) -> (date string=w443:string)  [unwired: 2 in, 1 out]
        n204 = local read "Summary"() -> (w446:T2)
        n205 = Bundle By Name(cluster=w446, "#user.lib VIs"=w445, "# of Unreviewed VIs (user.lib)"=w444, "Review Date(user.lib)"=w443, "# withoutCaller(user.lib)"=w442, "# of Modifed VIs (user.lib)"=w441) -> (w447:T2)
        n206 = local write "Summary"(w447) -> ()
        n207 = call <vilib>:"Add State(s) to Queue__jki_lib_state_machine.vi"("State(s) in (\"\")"=w465) -> ("States Out"=w464:string)  [unwired: 14 in]
      }
      frame "3rd Party: List Items" {
        # "List All The VIs in the Project\n(You can make a copy of, or modify, this frame)"
        n208 = Unbundle By Name(w479) -> ("Project Items.VIs In vi.lib"=w481:refnum<vi>[])
        n209 = control-ref of="Progress"() -> (w484:refnum<vi>)
        n210 = for {
          tunnel: w481 -> [w494] mode=indexing
          tunnel: w484 -> [w492]
          tunnel: [w487] -> w477 mode=indexing
          i -> [w491]
          n211 = property class="ProjectItem"(reference=w494) -> ("Name"=w488:string, "Path"=w490:path)  [unwired: 1 in, 2 out]
          n212 = Increment(x=w491) -> (x+1=w493:i32)
          n213 = property on="Property Node" class="Slide (strict)"(reference=w492, "Value"=w493) -> ()  [unwired: 1 in, 2 out]
          n214 = Path To String(path=w490) -> (string=w489:string)
          n215 = Build Array(w488, w489) -> (w487:string[])
        }
        n216 = Array Size(array=w481) -> (size(s)=w482:i32)
        n217 = To Double Precision Float(number=w482) -> (double precision float=w483:dbl)
        n218 = property on="Progress" class="Slide (strict)"("Scale.Maximum"=w483) -> ()  [unwired: 2 in, 2 out]
        n219 = Bundle By Name(cluster=w479, "3rd Party Member Data"=w477) -> (w478:T9)
        n220 = call <vilib>:"Add State(s) to Queue__jki_lib_state_machine.vi"("State(s) in (\"\")"=w486) -> ("States Out"=w485:string)  [unwired: 14 in]
      }
      frame "Project: Scan Complete" {
        # "Inform the User that the scan has been completed\n(You can make a copy of, or modify, this frame)"
        n221 = property on="Progress" class="Slide (strict)"("Caption.Text"="The Project Scan Has Been Completed.") -> ()  [unwired: 2 in, 2 out]
        n222 = call <vilib>:"Add State(s) to Queue__jki_lib_state_machine.vi"("State(s) in (\"\")"=w499) -> ("States Out"=w498:string)  [unwired: 14 in]
      }
      frame "Project: Get Project Info" {
        w504 = string[][] [] ("User.lib Member Data")
        # "List All The VIs in the Project\n(You can make a copy of, or modify, this frame)"
        n223 = Unbundle By Name(w512) -> ("Selected Project"=w510:refnum<vi>)
        n224 = property class="Project"(reference=w510, error in=w509) -> (error out=w508:errorcluster, "Name"=w502:string, "Path"=w507:path, "Description"=w500:string)  [unwired: 1 out]
        n225 = Strip Path(path=w507) -> (stripped path=w501:path)  [unwired: 1 out]
        n226 = Bundle By Name(cluster=w512, "Project Summary"=T8 {"Project Name"="", "Project Path"=path "", "# VIs in Project"=0, "# VIs Unreviewed"=0, "Date of Last Review"=timestamp(0 s since 1904-01-01), "# of VIs without Caller"=0, "Project Description"="", "# VIs Modified"=0}, "Project Items"=T7 {"VIs In Project"=[], "VIs In user.lib"=[], "VIs In vi.lib"=[]}, "Project Member Data"=w504, "User.lib Member Data"=w504, "3rd Party Member Data"=w504, "Unref Files"=path[] [], "Project Summary.Project Name"=w502, "Project Summary.Project Path"=w501, "Project Summary.Project Description"=w500) -> (w511:T9)
        n227 = call <vilib>:"Add State(s) to Queue__jki_lib_state_machine.vi"("State(s) in (\"\")"=w514) -> ("States Out"=w513:string)  [unwired: 14 in]
      }
      frame "Project: List Members" {
        w528 = "VI"  # Type
        w529 = TRUE ("ExcludeDependencies")
        # "List All The VIs in the Project\n(You can make a copy of, or modify, this frame)"
        n228 = Unbundle By Name(w526) -> ("Project Items"=w516:T7, "Selected Project"=w533:refnum<vi>)
        n229 = property class="Project"(reference=w533, error in=w532) -> (error out=w530:errorcluster, "My Computer"=w531:refnum<vi>)  [unwired: 1 out]
        n230 = invoke class="TargetItem" method="Get All Descendents"(reference=w531, error in=w530, "Type"=w528, "Exclude Dependencies"=FALSE ("ExcludeDependencies"), "ExcludeBuilds"=w529, "ExcludeTargets"=w529) -> (error out=w524:errorcluster, "All Descendents"=w520:refnum<vi>[])  [unwired: 1 in, 5 out]
        n231 = property on="Tab Control" class="TabCtl (strict)"("Val(Sgnl)"=T1."Summary" ("Value (Signaling)")) -> ()  [unwired: 2 in, 2 out]
        n232 = Array Size(array=w520) -> (size(s)=w522:i32)
        n233 = To Double Precision Float(number=w522) -> (double precision float=w523:dbl)
        n234 = control-ref of="Progress"() -> (w517:refnum<vi>)
        n235 = property on="Progress" class="Slide (strict)"("Scale.Maximum"=w523) -> ()  [unwired: 2 in, 2 out]
        n236 = property on="Progress" class="Slide (strict)"("Caption.Text"="Sorting Project Items By Location") -> ()  [unwired: 2 in, 2 out]
        n237 = call "Sort Project Items.vi"("Slide in"=w517, "Project Items"=w520, "Sorted VIs in"=w516) -> ("Sorted VIs out"=w519:T7)  [unwired: 8 in]
        n238 = Bundle By Name(cluster=w526, "Project Items"=w519) -> (w525:T9)
        n239 = call <vilib>:"Add State(s) to Queue__jki_lib_state_machine.vi"("State(s) in (\"\")"=w535, "State(s) at Back (\"\")"="Project: Get Member Info\nUser.lib:  Get Info\n3rd Party: List Items\nProject: Check Folder\nProject: Scan Complete" ("State")) -> ("States Out"=w534:string)  [unwired: 13 in]
      }
    }
  }
  n240 = Unbundle By Name(w2) -> ("Selected Project"=→"Selected Project Out":refnum<vi>)
